vi "Visualize_Tracks_Different_Colours-1.vi"(4 "[IN] Additional Index":i32, 5 "[IN] Delete Tracs":bool, 6 "error IN":errorcluster, 7 "[IN] Testing Frame":u32 min=24 max=58, 8 "[IN] Tracks":T2, 9 "[IN] LoG Pro-\ncessed Image":T1) -> (0 "error OUT":errorcluster, 3 "[OUT] Image with\nDisplacements":T1)   [LabVIEW 2017]
uses:
  <vilib>/vision/Image Controls.llb/IMAQ Image.ctl
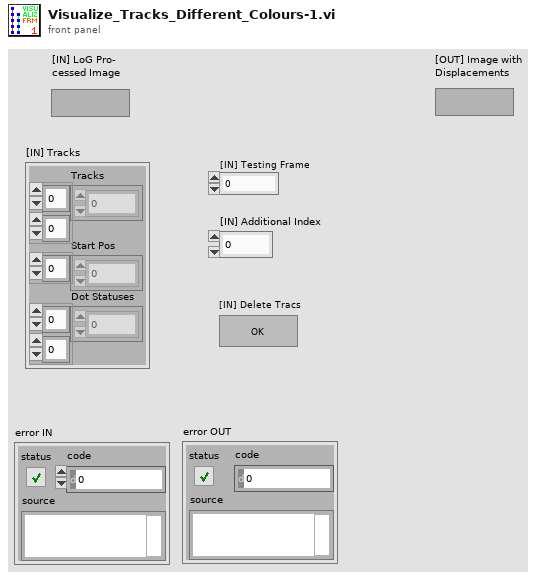
[diagram p1: front panel]
types:
  T1 = typedef "IMAQ Image.ctl" = refnum<image>
  T2 = cluster{"Tracks":dbl[][], "Start Pos":i32[], "Dot Statuses":i16[][]}
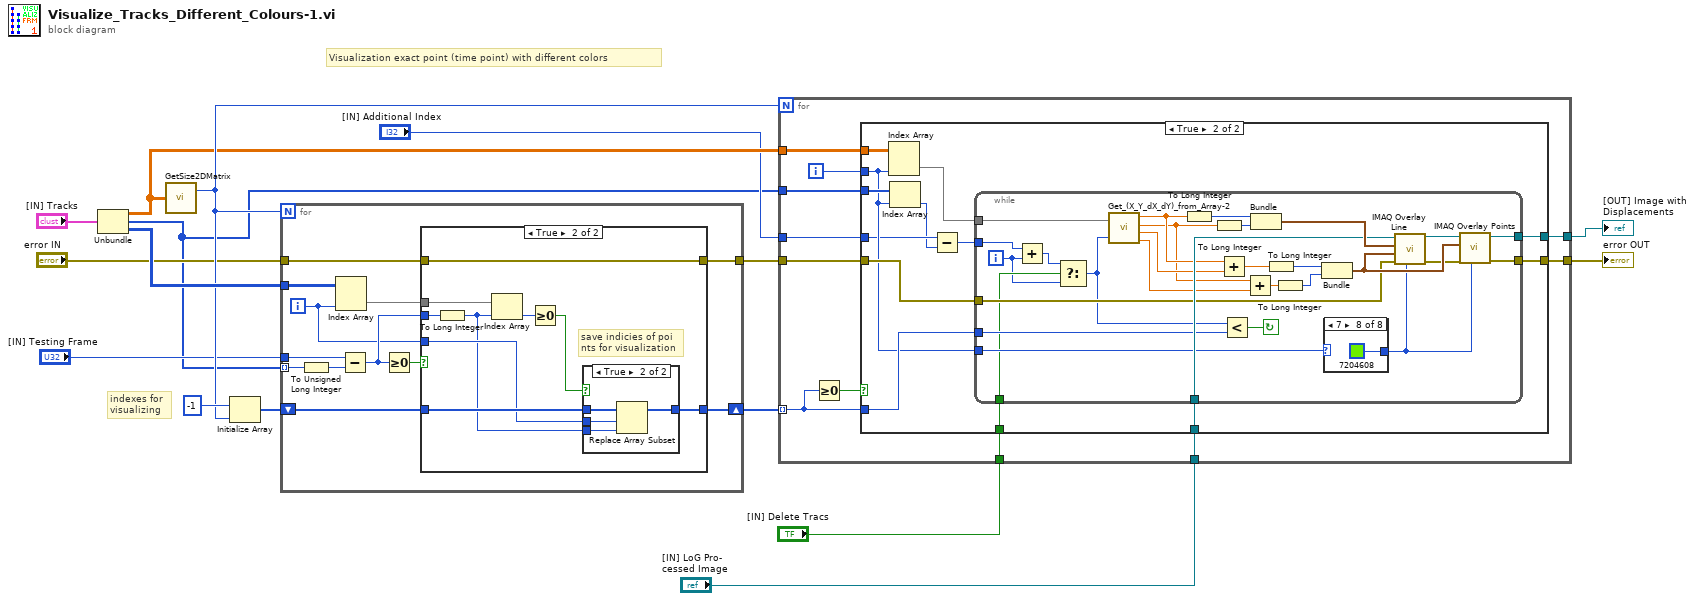
[diagram p0: block diagram]
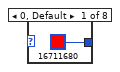
[diagram p3: hidden frame]
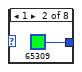
[diagram p4: hidden frame]
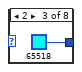
[diagram p5: hidden frame]
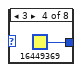
[diagram p6: hidden frame]
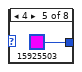
[diagram p7: hidden frame]
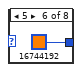
[diagram p8: hidden frame]
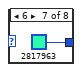
[diagram p9: hidden frame]
diagram:
  # "Visualization exact point (time point) with different colors"
  # "indexes for \nvisualizing"
  n1 = Unbundle("[IN] Tracks") -> ("Tracks"=w10:dbl[][], "Start Pos"=w1:i32[], "Dot Statuses"=w15:i16[][])
  n2 = call "GetSize2DMatrix.vi"("Array IN (2D)"=w10) -> ("# Cols"=w12:i32)  [unwired: 1 out]
  n3 = Initialize Array(-1 ("element"), w12) -> (w13:i32[])
  n4 = for {
    N: w12 -> [_]
    tunnel: w15 -> [w28]
    shift-right: [w19] -> w11
    shift-left: w13 -> [w21]
    tunnel: "[IN] Testing Frame" -> [w27]
    tunnel: w1 -> [w26] mode=indexing
    tunnel: "error IN" -> [w18]
    tunnel: [w17] -> w7
    i -> [w20]
    n5 = To Unsigned Long Integer(number=w26) -> (unsigned 32bit integer=w25:u32)
    n6 = Index Array(array=w28, index (col)=w20) -> (element=w23:i16[])  [unwired: 1 in]
    n7 = Subtract(x=w27, y=w25) -> (x-y=w22:u32)
    n8 = Greater Or Equal To 0?(x=w22) -> (x >= 0?=w24:bool)
    n9 = case shown="True" w24 {
      tunnel: w23 -> [_ w39]
      tunnel: w22 -> [_ w34]
      tunnel: w21 -> [w30 w36]
      tunnel: w20 -> [_ w35]
      tunnel: [w30 w33] -> w19
      tunnel: w18 -> [w29 w31]
      tunnel: [w29 w31] -> w17
      frame False {
      }
      frame True {
        # "save indicies of poi\nnts for visualization"
        n10 = To Long Integer(number=w34) -> (32bit integer=w32:i32)
        n11 = Index Array(array=w39, index=w32) -> (element=w38:i16)
        n12 = Greater Or Equal To 0?(x=w38) -> (x >= 0?=w37:bool)
        n13 = case shown="True" w37 {
          tunnel: w36 -> [w40 w44]
          tunnel: w35 -> [_ w43]
          tunnel: w32 -> [_ w42]
          tunnel: [w40 w41] -> w33
          frame False {
          }
          frame True {
            n14 = Replace Array Subset(array=w44, new element=w42, index=w43) -> (w41:i32[])
          }
        }
      }
    }
  }
  n15 = for {
    N: w12 -> [_]
    tunnel: w11 -> [w54] mode=indexing
    tunnel: w10 -> [w53]
    tunnel: "[IN] LoG Pro-\ncessed Image" -> [w51]
    tunnel: w7 -> [w50]
    tunnel: [w49] -> w5
    tunnel: [w48] -> w6
    tunnel: "[IN] Delete Tracs" -> [w47]
    tunnel: "[IN] Additional Index" -> [w46]
    tunnel: w1 -> [w45]
    i -> [w52]
    n16 = Greater Or Equal To 0?(x=w54) -> (x >= 0?=w55:bool)
    n17 = case shown="True" w55 {
      tunnel: w54 -> [_ w68]
      tunnel: w53 -> [_ w70]
      tunnel: w52 -> [_ w61]
      tunnel: w51 -> [w57 w67]
      tunnel: w50 -> [w56 w66]
      tunnel: [w57 w65] -> w49
      tunnel: [w56 w64] -> w48
      tunnel: w47 -> [_ w63]
      tunnel: w46 -> [_ w60]
      tunnel: w45 -> [_ w62]
      frame False {
      }
      frame True {
        n18 = Index Array(array=w70, index (col)=w61) -> (element=w69:dbl[])  [unwired: 1 in]
        n19 = Index Array(array=w62, index=w61) -> (element=w59:i32)
        n20 = Subtract(x=w60, y=w59) -> (x-y=w58:i32)
        n21 = while {
          tunnel: w69 -> [w98]
          tunnel: w68 -> [w78]
          tunnel: w67 -> [w87]
          tunnel: w66 -> [w82]
          tunnel: [w80] -> w65
          tunnel: [w79] -> w64
          tunnel: w61 -> [w76]
          tunnel: w63 -> [w75]
          tunnel: w58 -> [w73]
          i -> [w74]
          stop <- w77 continue-if-true
          n22 = Add(x=w73, y=w74) -> (x+y=w72:i32)
          n23 = Select(t=w72, s=w75, f=w74) -> (s? t:f=w71:i32)
          n24 = call "Get_(X_Y_dX_dY)_from_Array-2.vi"("(X,Y,dX,dY)"=w98, "Index of Displacement"=w71) -> ("X"=w86:dbl, "Y"=w84:dbl, "dX"=w85:dbl, "dY"=w83:dbl)
          n25 = To Long Integer(number=w86) -> (32bit integer=w89:i32)
          n26 = To Long Integer(number=w84) -> (32bit integer=w88:i32)
          n27 = Add(x=w86, y=w85) -> (x+y=w91:dbl)
          n28 = Less?(x=w71, y=w78) -> (x < y?=w77:bool)
          n29 = Add(x=w84, y=w83) -> (x+y=w93:dbl)
          n30 = Bundle(w89, w88) -> (w97:cluster{i32, i32})  [unwired: 1 in]
          n31 = To Long Integer(number=w91) -> (32bit integer=w90:i32)
          n32 = To Long Integer(number=w93) -> (32bit integer=w92:i32)
          n33 = Bundle(w90, w92) -> (w95:cluster{i32, i32})  [unwired: 1 in]
          n34 = case shown="7" w76 {
            tunnel: [u32 16711680 ("Color") u32 65309 ("Color") u32 65518 ("Color") u32 16449369 ("Color") u32 15925503 ("Color") u32 16744192 ("Color") u32 2817963 ("Color") u32 7204608 ("Color")] -> w81
            frame 0, Default {
            }
            frame 1 {
            }
            frame 2 {
            }
            frame 3 {
            }
            frame 4 {
            }
            frame 5 {
            }
            frame 6 {
            }
            frame 7 {
            }
          }
          n35 = call "IMAQ Overlay Line"("Color"=w81, "error in (no error)"=w82, "End Point"=w95, "Start Point"=w97, "Image"=w87) -> ("error out"=w94:errorcluster, "Image Out"=w96:T1)  [unwired: 5 in]
          n36 = call "IMAQ Overlay Points"("Color"=w81, "error in (no error)"=w94, "Point"=w95, "Image"=w96) -> ("error out"=w79:errorcluster, "Image Out"=w80:T1)  [unwired: 6 in]
        }
      }
    }
  }
  "error OUT" <- w6
  "[OUT] Image with\nDisplacements" <- w5
